vi "RTM - Remove Diagnostic Channels.vi"(8 "error in (no error)":errorcluster, 11 "Node Ptr":u64 format="%.0x") -> (0 "error out":errorcluster)   [LabVIEW 2016, in "UDP-Custom-Device System Explorer.lvlib"]
uses:
  UDP-Custom-Device System Explorer.lvlib
  Shared/Constants.vi
  <vilib>/NI VeriStand/Custom Device API/Custom Device API.lvlib
  Shared/UDP-Custom-Device Shared.lvlib
  <vilib>/NI Veristand/Custom Device API/Set Item Property (Boolean).vi
panel:
  in  "Tag":string
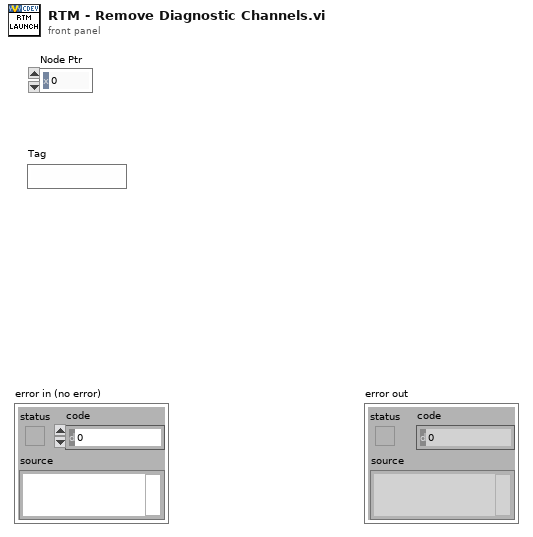
[diagram p1: front panel]
types:
  T1 = typedef "Custom Device API.lvlib/Custom Device Item Ref.ctl" = u64
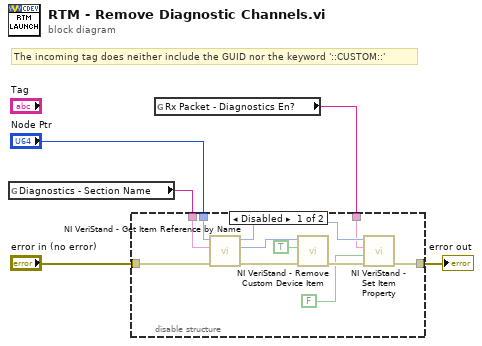
[diagram p0: block diagram]
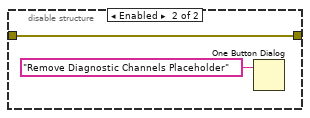
[diagram p2: hidden frame]
diagram:
  # "The incoming tag does neither include the GUID nor the keyword '::CUSTOM::'"
  n1 = global read "Constants.vi" "Diagnostics - Section Name"() -> (w3:string)
  n2 = global read "Constants.vi" "Rx Packet - Diagnostics En?"() -> (w1:string)
  n3 = disable-structure shown="Disabled" {
    disable-tunnel: "error in (no error)" -> [w16 w17]
    disable-tunnel: "Node Ptr" -> [w14 _]
    disable-tunnel: w3 -> [w13 _]
    disable-tunnel: [w10 w17] -> w2
    disable-tunnel: w1 -> [w8 _]
    frame Disabled {
      n4 = call <vilib>:"NI VeriStand - Get Item Reference by Name.vi"("error in (no error)"=w16, "Item Name"=w13, "Parent Ref in"=w14) -> ("error out"=w15:errorcluster, "Item Ref"=w12:T1, "Parent Ref out"=w9:T1)  [unwired: 5 in, 1 out]
      n5 = call <vilib>:"NI VeriStand - Remove Custom Device Item.vi"("error in (no error)"=w15, "Force Delete (F)"=TRUE, "Item Ref in"=w12) -> ("error out"=w11:errorcluster)  [unwired: 7 in, 1 out]
      n6 = call-poly <vilib>:"NI VeriStand - Set Item Property.vi"("error in (no error)"=w11, "Value"=FALSE, "Property Name"=w8, "Item Ref in"=w9) -> ("error out"=w10:errorcluster)  [unwired: 5 in, 2 out]
    }
    frame Enabled {
      n7 = One Button Dialog(message="Remove Diagnostic Channels Placeholder") -> ()  [unwired: 1 in, 1 out]
    }
  }
  "error out" <- w2
